vi "checkBeginHaltPlay.vi"(8 "error in (no error)":errorcluster, 10 "Game":refnum<class "Game.lvclass">, 11 "HaltPlay in":refnum<class "HaltPlay.lvclass">) -> (0 "error out":errorcluster, 2 "Boolean":bool, 3 "HaltPlay out":refnum<class "HaltPlay.lvclass">)   [LabVIEW 2020, in "HaltPlay.lvclass"]
uses:
  HaltPlay.lvclass
  Game_class/Game.lvclass
  Game_class/Game.lvclass/Game.ctl
  Events_class/Events.lvclass/Events.ctl
  Game_class/Read Referee.vi
  Game_class/Read EventsRef.vi
  Events_class/Read ball_out_of_vision.vi
  Referee_class/Referee.lvclass
  Events_class/Events.lvclass
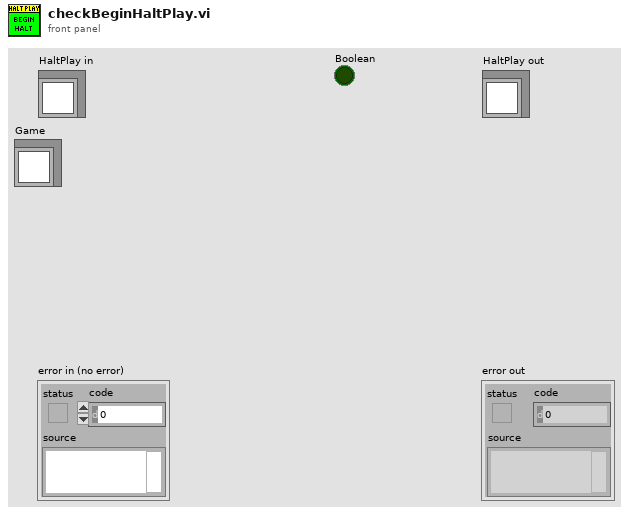
[diagram p1: front panel]
types:
  T1 = enum16{"AUTO", "GAME_ON", "STOP", "HALT", "KICKOFF", "FREE_BALL", "GOAL_KICK", "PENALTY_KICK", "FREE_KICK"}
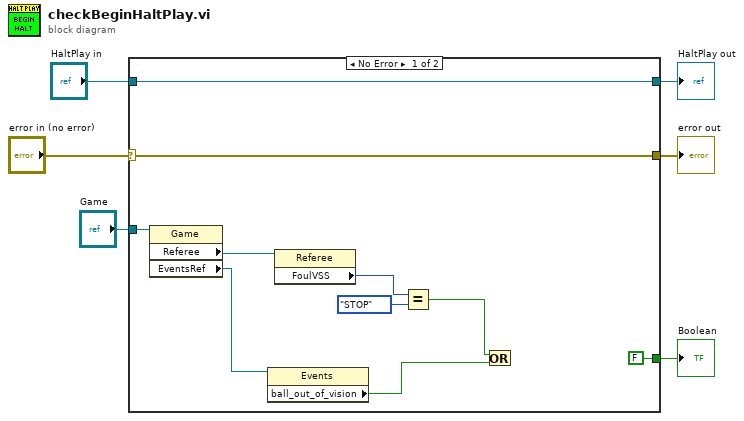
[diagram p0: block diagram]
diagram:
  n1 = case shown="No Error" "error in (no error)" {
    selector: "error in (no error)" -> [w15 w18]
    tunnel: [w15 w18] -> w5
    tunnel: [w16 w17] -> w3
    tunnel: "HaltPlay in" -> [w16 w17]
    tunnel: "Game" -> [w14 _]
    tunnel: [FALSE _] -> w1
    frame No Error {
      n2 = property class="Game"(reference=w14) -> ("Referee"=w13:refnum<class "Referee.lvclass">, "EventsRef"=w12:refnum<class "Events.lvclass">)  [unwired: 1 in, 2 out]
      n3 = property class="Events"(reference=w12) -> ("ball_out_of_vision"=w11:bool)  [unwired: 1 in, 2 out]
      n4 = property class="Referee"(reference=w13) -> ("FoulVSS"=w10:T1)  [unwired: 1 in, 2 out]
      n5 = Equal?(x=w10, y=T1."STOP") -> (x = y?=w9:bool)
      n6 = Or(x=w9, y=w11) -> ()  [unwired: 1 out]
    }
    frame Error {
    }
  }
  "error out" <- w5
  "HaltPlay out" <- w3
  "Boolean" <- w1
